vi "optionsAcq_spectrumType.vi"(8 "error in (no error)":errorcluster, 9 "readWrite":enum16{"read", "write"}(ring), 10 "spectrum channel type":T1, 11 "Thorlabs_OSA200_64 in":refnum<class "OSA200.lvclass">) -> (0 "error out":errorcluster, 2 "spectrum channel out":T1, 3 "Thorlabs_OSA200_64 out":refnum<class "OSA200.lvclass">)   [LabVIEW 2010, in "OSA200.lvclass"]
uses:
  OSA200.lvclass
  _misc/Thorlabs_FTS_misc.llb/channelType_spectrum.ctl
  OSA.lvclass
  OSA20X_misc.lvlib
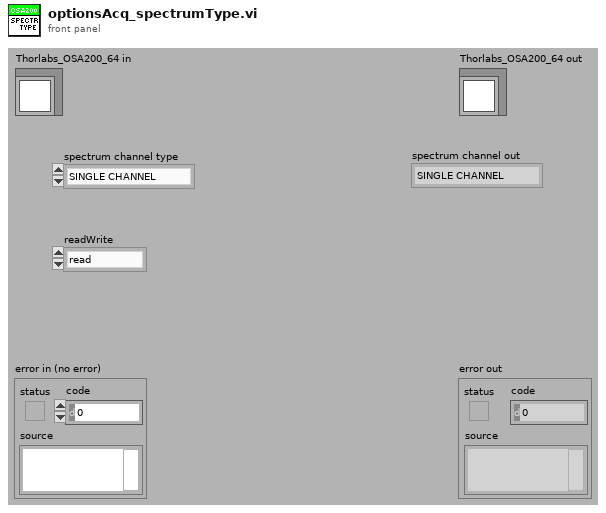
[diagram p1: front panel]
types:
  T1 = typedef "OSA20X_misc.lvlib/channelType_spectrum.ctl" = enum16{"SINGLE CHANNEL", "STICHED"}
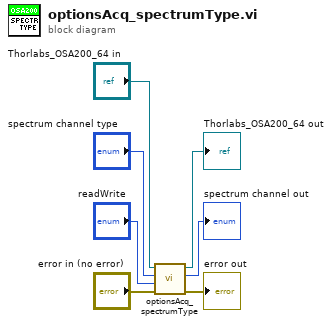
[diagram p0: block diagram]
diagram:
  n1 = call-parent "optionsAcq_spectrumType.vi"("error in (no error)"="error in (no error)", "readWrite"="readWrite", "spectrum channel type"="spectrum channel type", "Thorlabs_OSA_64 in"="Thorlabs_OSA200_64 in") -> ("error out"=→"error out":errorcluster, "spectrum channel out"=→"spectrum channel out":T1, "Thorlabs_OSA_64 out"=→"Thorlabs_OSA200_64 out":refnum<class "OSA200.lvclass">)  [unwired: 5 in]
